vi "循环发送CAN.vi"(8 "错误输入":errorcluster caption="错误输出") -> (0 "错误输出":errorcluster)   [LabVIEW 2020]
uses:
  Global_Variable/Global.vi
  Libraries/ZLG_CAN/CAN_CYCLE.vi
  Libraries/ZLG_CAN/ZLG_CAN.lvlib
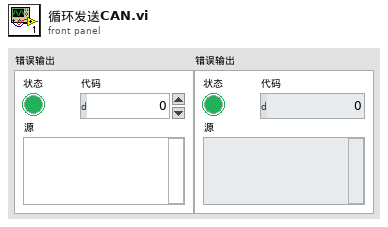
[diagram p1: front panel]
types:
  T1 = enum32{"Invalid", "Standard", "Closed", "Hidden", "Minimized", "Maximized"}
  T2 = cluster{"ID":u32, "帧类型":enum8{"标准帧", "扩展帧"}, "帧格式":enum16{"数据帧", "远程帧"}, "帧数据":string, "周期(ms)":u32}[]
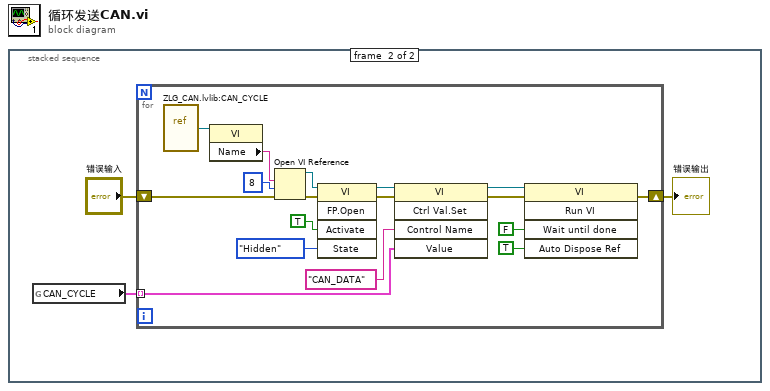
[diagram p0: block diagram]
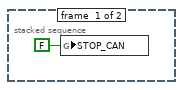
[diagram p2: hidden frame]
diagram:
  n1 = stacked-sequence {
    frame #0 {
      n2 = global write "Global.vi" "STOP_CAN"(FALSE ("STOP_CAN")) -> ()
    }
    frame #1 {
      n3 = global read "Global.vi" "CAN_CYCLE"() -> (w4:T2)
      n4 = for {
        tunnel: w4 -> [w15] mode=indexing
        shift-right: [w7] -> w2
        shift-left: "错误输入" -> [w18]
        n5 = vi-ref "ZLG_CAN.lvlib:CAN_CYCLE.vi"() -> (w21:refnum<vi>)
        n6 = property class="VI"(reference=w21) -> ("Name"=w20:string)  [unwired: 1 in, 2 out]
        n7 = Open VI Reference(vi path=w20, options=8 ("选项"), error in (no error)=w18) -> (vi reference=w17:refnum<vi>, error out=w13:errorcluster)  [unwired: 3 in]
        n8 = invoke class="VI" method="FP.Open"(reference=w17, error in=w13, "Activate"=TRUE ("激活？"), "State"=T1."Hidden" ("状态")) -> (reference out=w14:refnum<vi>, error out=w12:errorcluster)  [unwired: 1 in, 3 out]
        n9 = invoke class="VI" method="Ctrl Val.Set"(reference=w14, error in=w12, "Control Name"="CAN_DATA" ("控件名"), "Value"=w15) -> (reference out=w9:refnum<vi>, error out=w8:errorcluster)  [unwired: 1 in, 3 out]
        n10 = invoke class="VI" method="Run VI"(reference=w9, error in=w8, "Wait until done"=FALSE ("结束前等待"), "Auto Dispose Ref"=TRUE ("自动销毁引用")) -> (error out=w7:errorcluster)  [unwired: 1 in, 4 out]
      }
      "错误输出" <- w2
    }
  }
